vi "getEnumerationType.vi"(8 "error in (no error)":errorcluster, 11 "IEnumeration in":refnum<class "IEnumeration.lvclass">) -> (0 "error out":errorcluster, 2 "Enumeration Type out":refnum<class "IEnumerationType.lvclass">, 3 "IEnumeration out":refnum<class "IEnumeration.lvclass">)   [LabVIEW 2022 SP3, in "openDAQ.lvlib" / "daqCoreTypes.lvlib" / "IEnumeration.lvclass"]
uses:
  <instrlib>/openDAQ/Public/Classes/daqCoreTypes/IEnumeration/IEnumeration.lvclass
  C:/Program Files (x86)/National Instruments/LabVIEW 2022/instr.lib/openDAQ/Public/Classes/IBaseObject/IBaseObject.lvclass
  <instrlib>/openDAQ/Public/Classes/daqCoreTypes/IEnumerationType/IEnumerationType.lvclass
  <instrlib>/openDAQ/Public/Classes/IBaseObject/IBaseObject.lvclass/IBaseObject.ctl
  <instrlib>/openDAQ/Public/Classes/IBaseObject/Accessor/Write reference.vi
  <instrlib>/openDAQ/Public/Classes/IBaseObject/Accessor/Read reference.vi
  <instrlib>/openDAQ/Binaries/Windows/x86/copendaq32.dll
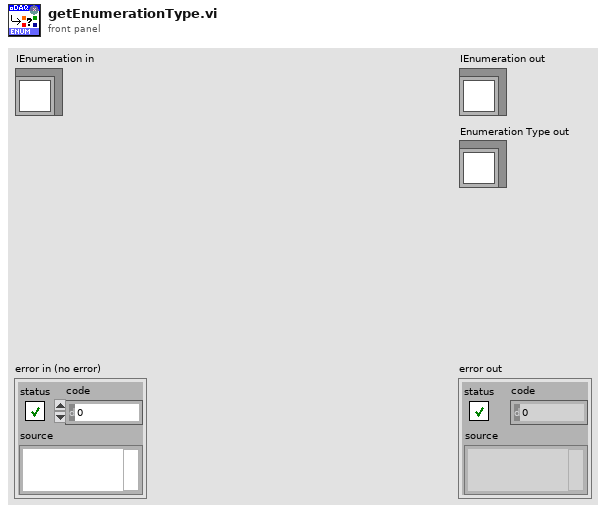
[diagram p1: front panel]
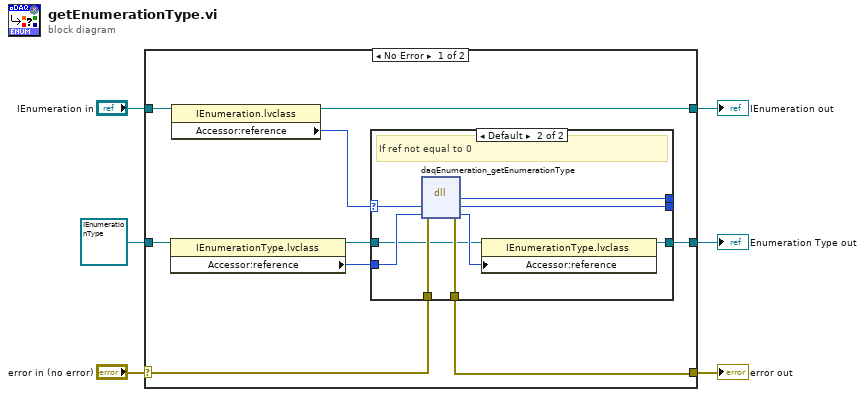
[diagram p0: block diagram]
diagram:
  n1 = case shown="No Error" "error in (no error)" {
    selector: "error in (no error)" -> [w10 w29]
    tunnel: [w8 w29] -> w5
    tunnel: [w13 w28] -> w3
    tunnel: "IEnumeration in" -> [w15 w28]
    tunnel: refnum<class "IEnumerationType.lvclass"> refnum -> [w9 w27]
    tunnel: [w7 w27] -> w1
    frame No Error {
      n2 = property class="IEnumerationType.lvclass"(reference=w9) -> (reference out=w12:refnum<class "IEnumerationType.lvclass">, "Accessor:reference"=w11:i64)  [unwired: 1 in, 1 out]
      n3 = property class="IEnumeration.lvclass"(reference=w15) -> (reference out=w13:refnum<class "IEnumeration.lvclass">, "Accessor:reference"=w14:i64)  [unwired: 1 in, 1 out]
      n4 = case shown="Default" w14 {
        selector: w14 -> [_ w24]
        tunnel: w10 -> [w16 w25]
        tunnel: w12 -> [w17 w18]
        tunnel: [w17 w20] -> w7
        tunnel: [_ w23] -> _
        tunnel: w11 -> [_ w21]
        tunnel: [_ w22] -> _
        tunnel: [w16 w19] -> w8
        frame 0 {
        }
        frame Default {
          # "If ref not equal to 0"
          n5 = dll-call lib="C:/Program Files (x86)/National Instruments/LabVIEW 2022/instr.lib/openDAQ/Binaries/Windows/x86/copendaq*.*" fn="daqEnumeration_getEnumerationType"(error in=w25, "enum"=w24, "type"=w21) -> (error out=w19:errorcluster, "return type"=w23:u32, "enum"=w22:i64, "type"=w26:i64)  [unwired: 2 in, 1 out]
          n6 = property class="IEnumerationType.lvclass"(reference=w18, "Accessor:reference"=w26) -> (reference out=w20:refnum<class "IEnumerationType.lvclass">)  [unwired: 1 in, 1 out]
        }
      }
    }
    frame Error {
    }
  }
  "error out" <- w5
  "IEnumeration out" <- w3
  "Enumeration Type out" <- w1
